vi "email_callback.vi"(8 "entrée d'erreur":errorcluster caption="entrée d'erreur (pas d'erreur)") -> (0 "error out":errorcluster caption="sortie d'erreur")   [LabVIEW 2020]
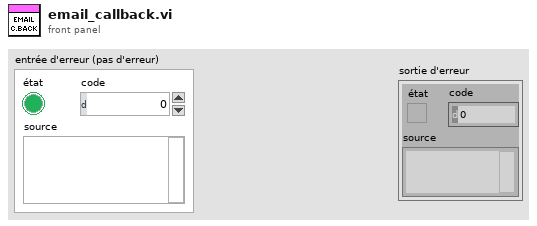
[diagram p1: front panel]
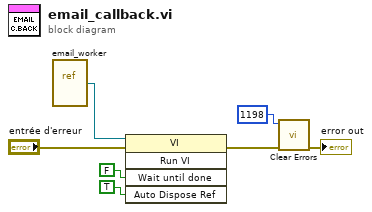
[diagram p0: block diagram]
diagram:
  n1 = vi-ref "email_worker.vi"() -> (w2:refnum<vi>)
  n2 = invoke class="VI" method="Run VI"(reference=w2, error in="entrée d'erreur", "Wait until done"=FALSE ("Attendre la fin"), "Auto Dispose Ref"=TRUE ("Supprimer la référence automatiquement")) -> (error out=w6:errorcluster)  [unwired: 1 in, 4 out]
  n3 = call <vilib>:"Clear Errors.vi"("error in (no error)"=w6, "specific error code to clear (0: all)"=1198) -> ("error out"=→"error out":errorcluster)  [unwired: 4 in, 1 out]
